vi "Griddy State Machine.vi"(6 "Griddy Started?":bool, 7 "Wrist":T1, 10 "Cascade":T1, 11 "Griddy Parameters":cluster{"Griddy Command":T6, "Flip Wrist?":bool}) -> (2 "Current Time":u32, 3 "Is Finished?":bool)   [LabVIEW 2020]
uses:
  Typedefs/Teleop Manipulator Commands.ctl
  <vilib>/Rock Robotics/WPI/MotorControl/WPI_MotorControlDeviceRef.ctl
  <vilib>/Rock Robotics/WPI/MotorControl/WPI_MotorControlType.ctl
  <vilib>/Rock Robotics/SystemInterfaces/DIO/FPGA_DIOPWMChannel.ctl
  <vilib>/Rock Robotics/WPI/PWM/WPI_PWMDeadband.ctl
  <vilib>/Rock Robotics/SystemInterfaces/DIO/FPGA_DIOChannel.ctl
  Typedefs/Manipulator State.ctl
  <vilib>/Rock Robotics/WPI/ThirdParty/REV Robotics/REVLib/Typedef/Spark MAX Control Type.ctl
  e17cb540-cf00-4f2d-b5e7-f53172b3d7b0.vi
  Framework/Robot Global Data.vi
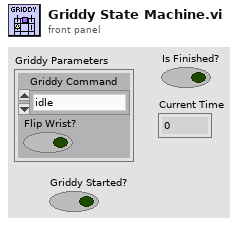
[diagram p1: front panel]
types:
  T1 = typedef "WPI_MotorControlDeviceRef.ctl" = cluster{"DeviceStatus":errorcluster, "Type":T2, "PWM":cluster{"PWM Channel":T3, "DeadBand":T4}, "CAN":cluster{"Device Number":u8, "SetOutput VI Ref":variant, "GetOutput VI Ref":variant, "Enable VI Ref":variant, "Disable VI Ref":variant, "Data":variant}, "Invert":bool, "DIO PWM":cluster{"PWM \"Enable\" Channel":T3, "DIOChannel":T5, "PWM Rate":dbl}}
  T2 = typedef "WPI_MotorControlType.ctl" = enum16{"PWM", "CAN", "DIO PWM"}
  T3 = typedef "FPGA_DIOPWMChannel.ctl" = enum8{"PWM 0", "PWM 1", "PWM 2", "PWM 3", "PWM 4", "PWM 5", "PWM 6", "PWM 7", "PWM 8", "PWM 9", "PWM MXP 0", "PWM MXP 1", "PWM MXP 2", "PWM MXP 3", "PWM MXP 4", "PWM MXP 5", "PWM MXP 6", "PWM MXP 7", "PWM MXP 8", "PWM MXP 9", "Invalid"}
  T4 = typedef "WPI_PWMDeadband.ctl" = cluster{"Name":string, "maxPositivePwm":i32, "minPositivePwm":i32, "centerPwm":i32, "maxNegativePwm":i32, "minNegativePwm":i32, "angularRange":u16}
  T5 = typedef "FPGA_DIOChannel.ctl" = enum8{"DIO 0", "DIO 1", "DIO 2", "DIO 3", "DIO 4", "DIO 5", "DIO 6", "DIO 7", "DIO 8", "DIO 9", "DIO MXP 0", "DIO MXP 1", "DIO MXP 2", "DIO MXP 3", "DIO MXP 4", "DIO MXP 5", "DIO MXP 6", "DIO MXP 7", "DIO MXP 8", "DIO MXP 9", "DIO MXP 10", "DIO MXP 11", "DIO MXP 12", "DIO MXP 13", "DIO MXP 14", "DIO MXP 15", "SPI Port CS1", "SPI Port CS2", "SPI Port CS3", "SPI Port MISO", "SPI Port MOSI", "Invalid"}
  T6 = typedef "Teleop Manipulator Commands.ctl" = enum16{"idle", "intake cone sideways", "intake cone upright", "intake cone feeder", "intake cube feeder", "intake cube", "score low cone", "score low cube", "score mid cone", "score mid cube", "score high cone", "score high cube", "score mid cone up"}
  T7 = typedef "Spark MAX Control Type.ctl" = enum16{"Percent VBus", "Voltage", "Velocity", "Position", "Smart Motion", "Current", "Smart Velocity"}
  T8 = typedef "Manipulator State.ctl" = enum16{"Wrist Safety", "Cascade", "Wrist Final", "Finished"}
  T9 = cluster{"Safe Wrist Position":dbl, "Margin of Error":cluster{"Safety Wrist Margin":dbl, "Cascade Margin":dbl, "Final Wrist Margin":dbl}, "grid-dy":cluster{"Griddy Preset":string, "cascade pos":dbl, "wrist pos":dbl, "Overrides":cluster{"Margin of Error Overrides":cluster{"Safety Wrist Margin":dbl, "Cascade Margin":dbl, "Final Wrist Margin":dbl}, "Override?":bool}}[]}
  T10 = cluster{"Safety Wrist Margin":dbl, "Cascade Margin":dbl, "Final Wrist Margin":dbl}
  T11 = cluster{"Griddy Preset":string, "cascade pos":dbl, "wrist pos":dbl, "Overrides":cluster{"Margin of Error Overrides":cluster{"Safety Wrist Margin":dbl, "Cascade Margin":dbl, "Final Wrist Margin":dbl}, "Override?":bool}}[]
  T12 = cluster{"Griddy Preset":string, "cascade pos":dbl, "wrist pos":dbl, "Overrides":cluster{"Margin of Error Overrides":cluster{"Safety Wrist Margin":dbl, "Cascade Margin":dbl, "Final Wrist Margin":dbl}, "Override?":bool}}
  T13 = cluster{"Margin of Error Overrides":cluster{"Safety Wrist Margin":dbl, "Cascade Margin":dbl, "Final Wrist Margin":dbl}, "Override?":bool}
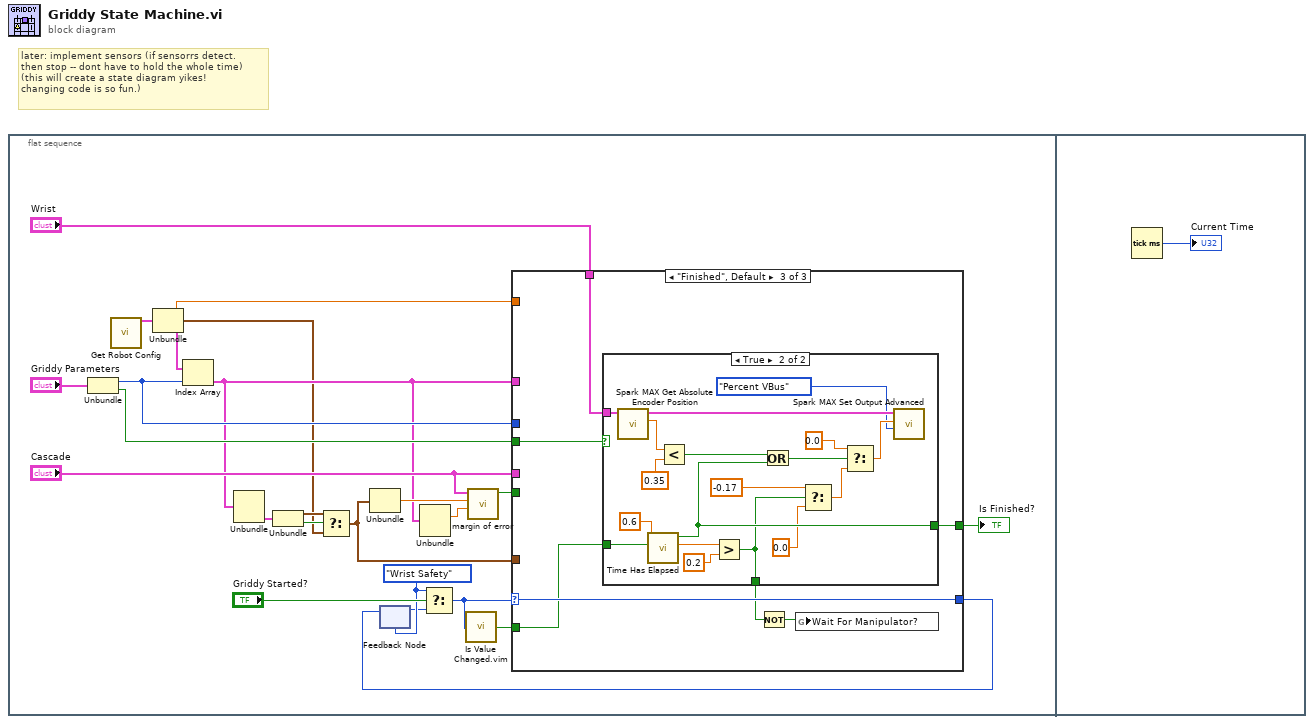
[diagram p0: block diagram]
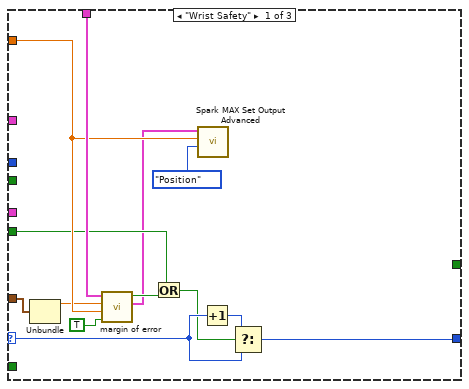
[diagram p2: hidden frame]
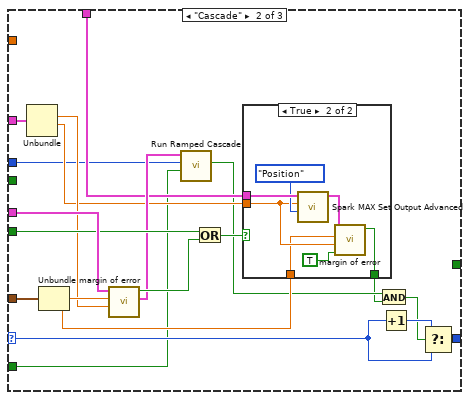
[diagram p3: hidden frame]
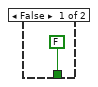
[diagram p4: hidden frame]
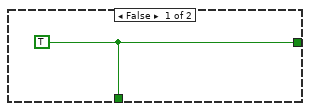
[diagram p5: hidden frame]
diagram:
  # "later: implement sensors (if sensorrs detect.\nthen stop -- dont have to hold the whole time)\n(this will create a state diagram yikes! \nchanging code is so fun.)"
  n1 = flat-sequence {
    frame #0 {
      w18 = Manipulator_State."Wrist Safety"
      n2 = Unbundle("Griddy Parameters") -> ("Griddy Command"=w10:T6, "Flip Wrist?"=w24:bool)
      n3 = call "Get Robot Config.vi"() -> ("Manipulator Config"=w9:T9)  [unwired: 12 in, 7 out]
      n4 = Unbundle(w9) -> ("Safe Wrist Position"=w13:dbl, "Margin of Error"=w2:T10, "grid-dy"=w15:T11)
      n5 = Index Array(array=w15, index=w10) -> (element=w6:T12)
      n6 = Unbundle(w6) -> ("Overrides"=w5:T13)  [unwired: 3 out]
      n7 = Unbundle(w5) -> ("Margin of Error Overrides"=w3:T10, "Override?"=w4:bool)
      n8 = Select(t=w3, s=w4, f=w2) -> (s? t:f=w1:T10)
      n9 = Unbundle(w1) -> ("Cascade Margin"=w16:dbl)  [unwired: 2 out]
      n10 = feedback #1(w18) -> (w17:T8)
      n11 = Unbundle(w6) -> ("cascade pos"=w21:dbl)  [unwired: 3 out]
      n12 = Select(t=w18, s="Griddy Started?", f=w17) -> (s? t:f=w8:T8)
      n13 = call "Is Value Changed.vim"("value"=w8) -> ("changed or first call?"=w7:bool)
      n14 = call "margin of error.vi"("setpoint"=w21, "margin of error"=w16, "Motor In"="Cascade") -> ("In Range?"=w14:bool)  [unwired: 7 in, 1 out]
      n15 = case shown="\"Finished\", Default" w8 {
        selector: w8 -> [w34 w56 w70]
        tunnel: w6 -> [_ w53 _]
        tunnel: [w33 w55 w70] -> w22
        tunnel: "Wrist" -> [w37 w45 w71]
        tunnel: "Cascade" -> [_ w54 _]
        tunnel: w13 -> [w36 _ _]
        tunnel: w14 -> [w31 w51 _]
        tunnel: w1 -> [w30 w50 _]
        tunnel: w24 -> [_ _ w72]
        tunnel: [_ _ w67] -> w12
        tunnel: w10 -> [_ w42 _]
        tunnel: w7 -> [_ w41 w68]
        frame "Wrist Safety" {
          n16 = Unbundle(w30) -> ("Safety Wrist Margin"=w29:dbl)  [unwired: 2 out]
          n17 = call "margin of error.vi"("Wrist Motor?"=TRUE, "setpoint"=w36, "margin of error"=w29, "Motor In"=w37) -> ("Motor Out"=w28:T1, "In Range?"=w32:bool)  [unwired: 6 in]
          n18 = Or(x=w31, y=w32) -> (x .or. y?=w26:bool)
          n19 = call <vilib>:"Spark MAX Set Output Advanced.vi"("Control Mode"=Spark_MAX_Control_Type."Position", "Setpoint"=w36, "MotorControlDevRef"=w28) -> ()  [unwired: 7 in, 2 out]
          n20 = Increment(x=w34) -> (x+1=w35:T8)
          n21 = Select(t=w35, s=w26, f=w34) -> (s? t:f=w33:T8)
        }
        frame "Cascade" {
          n22 = Unbundle(w53) -> ("cascade pos"=w47:dbl, "wrist pos"=w46:dbl)  [unwired: 2 out]
          n23 = Unbundle(w50) -> ("Cascade Margin"=w49:dbl, "Final Wrist Margin"=w43:dbl)  [unwired: 1 out]
          n24 = call "margin of error.vi"("setpoint"=w47, "margin of error"=w49, "Motor In"=w54) -> ("Motor Out"=w48:T1, "In Range?"=w52:bool)  [unwired: 7 in]
          n25 = call "Run Ramped Cascade.vi"("Reset?"=w41, "Griddy Command"=w42, "Cascade In"=w48) -> ("Finished?"=w40:bool)  [unwired: 7 in, 1 out]
          n26 = Or(x=w51, y=w52) -> (x .or. y?=w44:bool)
          n27 = case shown="True" w44 {
            tunnel: w46 -> [_ w62]
            tunnel: w45 -> [_ w65]
            tunnel: w43 -> [_ w61]
            tunnel: [FALSE ("In Range?") w60] -> w39
            frame False {
            }
            frame True {
              n28 = call <vilib>:"Spark MAX Set Output Advanced.vi"("Control Mode"=Spark_MAX_Control_Type."Position", "Setpoint"=w62, "MotorControlDevRef"=w65) -> ("MotorControlDevRef"=w63:T1)  [unwired: 7 in, 1 out]
              n29 = call "margin of error.vi"("Wrist Motor?"=TRUE, "setpoint"=w62, "margin of error"=w61, "Motor In"=w63) -> ("In Range?"=w60:bool)  [unwired: 6 in, 1 out]
            }
          }
          n30 = And(x=w40, y=w39) -> (x .and. y?=w38:bool)
          n31 = Increment(x=w56) -> (x+1=w57:T8)
          n32 = Select(t=w57, s=w38, f=w56) -> (s? t:f=w55:T8)
        }
        frame "Finished", Default {
          n33 = case shown="True" w72 {
            tunnel: w71 -> [_ w89]
            tunnel: [w73 w77] -> w67
            tunnel: w68 -> [_ w81]
            tunnel: [w73 w76] -> w66
            frame False {
              w73 = TRUE
            }
            frame True {
              n34 = call <vilib>:"Spark MAX Get Absolute Encoder Position.vi"("MotorControlDeviceRef in"=w89) -> ("Position"=w91:dbl, "MotorControlDeviceRef out"=w88:T1)  [unwired: 7 in, 2 out]
              n35 = call "Time Has Elapsed.vi"("Reset?"=w81, "Delay"=0.6) -> ("Elapsed Time"=w80:dbl, "Elapsed Time Passed?"=w77:bool)  [unwired: 8 in]
              n36 = Less?(x=w91, y=0.35) -> (x < y?=w84:bool)
              n37 = Greater?(x=w80, y=0.2) -> (0:w76:bool)
              n38 = Or(x=w84, y=w77) -> (x .or. y?=w83:bool)
              n39 = Select(t=-0.17, s=w76, f=0.0) -> (s? t:f=w78:dbl)
              n40 = Select(t=0.0, s=w83, f=w78) -> (s? t:f=w87:dbl)
              n41 = call <vilib>:"Spark MAX Set Output Advanced.vi"("Control Mode"=Spark_MAX_Control_Type."Percent VBus", "Setpoint"=w87, "MotorControlDevRef"=w88) -> ()  [unwired: 7 in, 2 out]
            }
          }
          n42 = Not(x=w66) -> (.not. x?=w69:bool)
          n43 = global write "Robot Global Data.vi" "Wait For Manipulator?"(w69) -> ()
        }
      }
      "Is Finished?" <- w12
      n44 = feedback-in #1(w22) -> ()
    }
    frame #1 {
      n45 = Tick Count (ms)() -> (millisecond timer value=→"Current Time":u32)
    }
  }
